vi "Ref Ctrl.vi"(5 "Offset":refnum<class "Offset.lvclass"> caption="Offset (None)", 6 "Size":refnum<class "Size.lvclass"> caption="Size (Unchanged)", 7 "Alignment":T1={"Horizontal"=enum."Center", "Vertical"=enum."Center"} caption="Alignment (Center, Center)", 8 "Error In":errorcluster, 10 "Ref Ctrl":refnum<vi>) -> (0 "Error Out":errorcluster, 3 "Ref Ctrl Out":refnum<class "Ref Ctrl.lvclass">)   [LabVIEW 2020, in "Panel.lvlib" / "Ref Ctrl.lvclass"]
doc: "Constructs a window positioner that will use a control's screen position as an anchor.\n\n<B>Ref Ctl:</B> Sets the control to use as a reference.\n<B>Alignment:</B> Set the type of alignment\n<B>Offset:</B> Input Offset object.\n<B>Size:</B> Display Size object.\n<B>Error In:</B> Describes error conditions that occur before this node runs.\n\n<B>Ref Ctl Out:</B> Ref Ctrl object.\n<B>Error Out:</B> Contains error information.\n----\nPlease see the following web address for additional documentation and tutorial information:\nhttp://www.mooregoodideas.com/mgi-panel-manager/\n\nAuthor: Derek Trepanier\n\nCopyright (c) 2018, Moore Good Ideas, Inc.\n\nAll rights reserved.\n\nRedistribution and use in source and binary forms, with or without modification, are permitted provided that the following conditions are met:\n\n * Redistributions of source code must retain the above copyright notice, this list of conditions and the following disclaimer.\n * Redistributions in binary form must reproduce the above copyright notice, this list of conditions and the following disclaimer in the documentation and/or other materials provided with the distribution.\n * Neither the name of Moore Good Ideas, Inc. nor the names of its contributors may be used to endorse or promote products derived from this software without specific prior written permission.\n\nTHIS SOFTWARE IS PROVIDED BY THE COPYRIGHT HOLDERS AND CONTRIBUTORS \"AS IS\" AND ANY EXPRESS OR IMPLIED WARRANTIES, INCLUDING, BUT NOT LIMITED TO, THE IMPLIED WARRANTIES OF MERCHANTABILITY AND FITNESS FOR A PARTICULAR PURPOSE ARE DISCLAIMED. IN NO EVENT SHALL THE COPYRIGHT OWNER OR CONTRIBUTORS BE LIABLE FOR ANY DIRECT, INDIRECT, INCIDENTAL, SPECIAL, EXEMPLARY, OR CONSEQUENTIAL DAMAGES (INCLUDING, BUT NOT LIMITED TO, PROCUREMENT OF SUBSTITUTE GOODS OR SERVICES; LOSS OF USE, DATA, OR PROFITS; OR BUSINESS INTERRUPTION) HOWEVER CAUSED AND ON ANY THEORY OF LIABILITY, WHETHER IN CONTRACT, STRICT LIABILITY, OR TORT (INCLUDING NEGLIGENCE OR OTHERWISE) ARISING IN ANY WAY OUT OF THE USE OF THIS SOFTWARE, EVEN IF ADVISED OF THE POSSIBILITY OF SUCH DAMAGE."
uses:
  <vilib>/MGI/Panel Manager/Panel/Window Position/Reference Position/Ref Ctrl/Ref Ctrl.lvclass
  C:/Program Files/National Instruments/LabVIEW 2020/vi.lib/MGI/Panel Manager/Panel/Window Position/Reference Position/Reference Position.lvclass
  <vilib>/MGI/Panel Manager/Panel/Window Position/Reference Position/Offset/Offset.lvclass
  <vilib>/MGI/Panel Manager/Panel/Window Position/Reference Position/Alignment.ctl
  <vilib>/MGI/Panel Manager/Panel/Window Position/Reference Position/Horizontal Alignment.ctl
  <vilib>/MGI/Panel Manager/Panel/Window Position/Reference Position/Vertical Alignment.ctl
  <vilib>/MGI/Panel Manager/Panel/Window Position/Reference Position/Size/Size.lvclass
  <vilib>/MGI/Panel Manager/Panel/Window Position/Reference Position/Ref Ctrl/Ref Ctrl.lvclass/Ref Ctrl.ctl
  <vilib>/MGI/Panel Manager/Panel/Window Position/Reference Position/Reference Position.lvclass
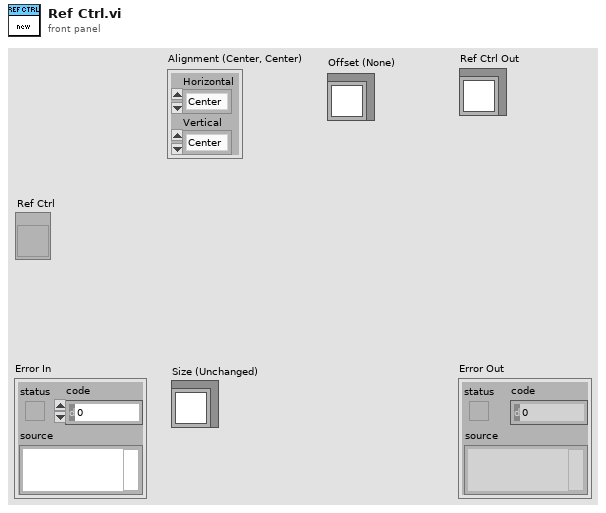
[diagram p1: front panel]
types:
  T1 = typedef "Panel.lvlib/Reference Position.lvclass/Alignment.ctl" = cluster{"Horizontal":T2, "Vertical":T3}
  T2 = typedef "Panel.lvlib/Reference Position.lvclass/Horizontal Alignment.ctl" = enum16{"Left", "Center", "Right"}
  T3 = typedef "Panel.lvlib/Reference Position.lvclass/Vertical Alignment.ctl" = enum16{"Top", "Center", "Bottom"}
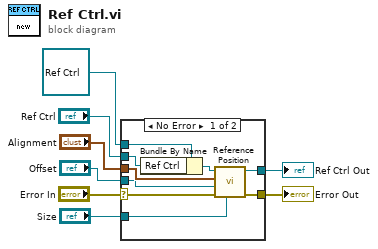
[diagram p0: block diagram]
diagram:
  n1 = case shown="No Error" "Error In" {
    selector: "Error In" -> [w13 w19]
    tunnel: [w12 w19] -> w7
    tunnel: [w14 w18] -> w5
    tunnel: refnum<class "Ref Ctrl.lvclass"> refnum ("Ref VI in") -> [w17 w18]
    tunnel: "Ref Ctrl" -> [w15 _]
    tunnel: "Alignment" -> [w11 _]
    tunnel: "Offset" -> [w10 _]
    tunnel: "Size" -> [w9 _]
    frame No Error {
      n2 = Bundle By Name(cluster=w17, "Ref Ctrl"=w15) -> (w16:refnum<class "Ref Ctrl.lvclass">)
      n3 = call <vilib>:"Reference Position.vi"("Size"=w9, "error in (no error)"=w13, "Offset"=w10, "Alignment"=w11, "Reference Position in"=w16) -> ("error out"=w12:errorcluster, "Reference Position out"=w14:refnum<class "Ref Ctrl.lvclass">)  [unwired: 5 in]
    }
    frame Error {
    }
  }
  "Error Out" <- w7
  "Ref Ctrl Out" <- w5
